vi "rqcBob Configure Window.vi"(8 "error in":errorcluster, 10 "window.config":T1={"window.open"=0, "window.close"=1820}, 11 "FPGA reference in":refnum<k20>) -> (0 "error out":errorcluster, 3 "FPGA reference out":refnum<k20>)   [LabVIEW 2019]
uses:
  FPGA/rqcBob/Custom Controls/rqcBob Window Config.ctl
  <vilib>/Utility/error.llb/Error Cluster From Error Code.vi
  <vilib>/rvi/errors/niLvFpgaAdjustHostInterfaceError.vi
  <vilib>/rvi/interface/nirviReadWriteControl/nirviReadWriteControl.xnode
  NiFpgaLv.dll
  <vilib>/rvi/interface/Simulation/niFpgaSimulationCallBeginRW.vi
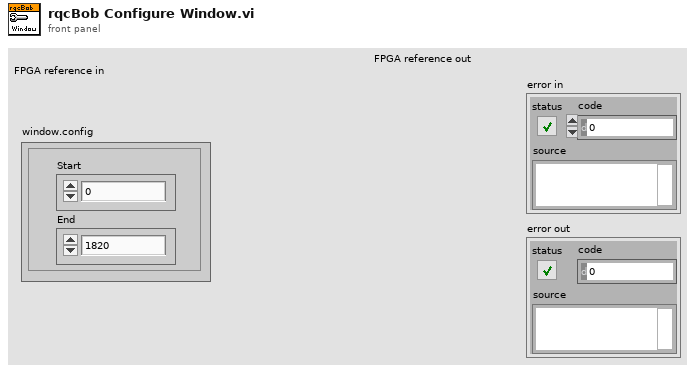
[diagram p1: front panel]
types:
  T1 = typedef "rqcBob Window Config.ctl" = cluster{"window.open":u16, "window.close":u16}
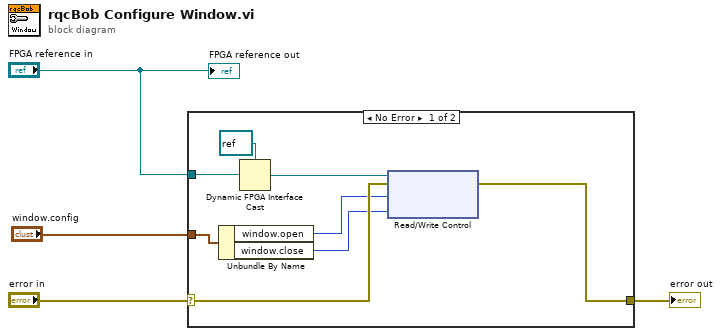
[diagram p0: block diagram]
diagram:
  n1 = case shown="No Error" "error in" {
    selector: "error in" -> [w12 w13]
    tunnel: [w11 w13] -> w2
    tunnel: "FPGA reference in" -> [w9 _]
    tunnel: "window.config" -> [w7 _]
    frame No Error {
      n2 = Unbundle By Name(w7) -> ("window.open"=w6:u16, "window.close"=w5:u16)
      n3 = Dynamic FPGA Interface Cast(Session In=refnum<k20> refnum ("FPGA Interface"), Type=w9) -> (Session Out=w8:refnum<k20>)
      n4 = xnode "Read/Write Control"("FPGA VI Reference In"=w8, "error in"=w12, "window.open"=w6, "window.close"=w5) -> ("error out"=w11:errorcluster)  [unwired: 1 out]
    }
    frame Error {
    }
  }
  "error out" <- w2
  "FPGA reference out" <- "FPGA reference in"
